vi "Check Finish Game.vi"(5 "Packed refs":T1, 7 "Game Result":refnum<vi>, 8 "error in (no error)":errorcluster, 11 "Board Game in":refnum<class "Board Game.lvclass">) -> (0 "error out":errorcluster, 1 "Finish Game?":bool, 3 "Board Game out":refnum<class "Board Game.lvclass">)   [LabVIEW 2021, in "Board Game.lvclass"]
uses:
  Board Game.lvclass
  Application/Packed Refs.ctl
  GameEl_class/private/Enum Direction.ctl
  Board Game.lvclass/Board Game.ctl
  Snake_class/Snake.lvclass/Snake.ctl
  GameEl_class/GameEl.lvclass/GameEl.ctl
  Imposible_Snake_v2/LVApp/Modules/Sound Manager/Typedefs/Sound Effects.ctl
  Game Result.ctl
  Snake_class/Read Bomb Crash.vi
  Snake_class/Read Star.vi
  GameEl_class/Read position.vi
  Snake_class/Read Snake Head.vi
  Snake_class/Snake.lvclass
  C:/Users/poche/Programs/LabVIEW/imposible snake/GameEl_class/GameEl.lvclass
  Imposible_Snake_v2/LVApp/Modules/Sound Manager/Sound Manager.lvlib
  GameEl_class/GameEl.lvclass
  Application/Game.lvclass
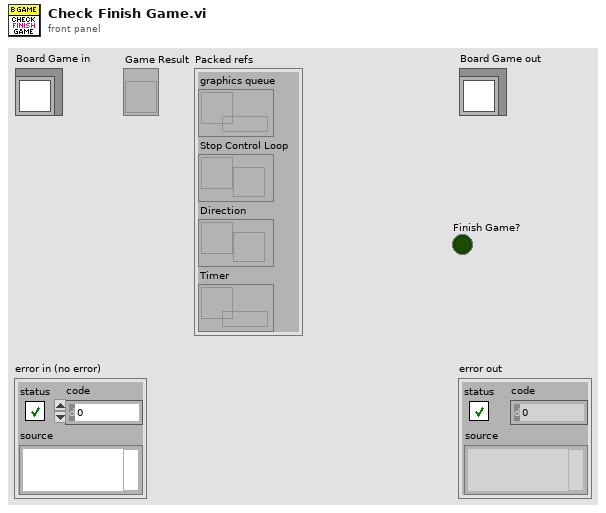
[diagram p1: front panel]
types:
  T1 = typedef "Game.lvclass/Packed Refs.ctl" = cluster{"graphics queue":refnum<queue>, "Stop Control Loop":refnum<user-event>, "Direction":refnum<notifier>, "Timer":refnum<data-value>}
  T2 = typedef "Sound Manager.lvlib/Sound Effects.ctl" = enum16{"Bomb In", "Bomb Out", "Bomb Touched", "Game Over", "Victory", "Eat", "10 Fruits", "Eat2", "Eat3", "Eat4", "MaxShield", "Shield", "10p", "Grape In", "Grape Out", "20p", "30p", "40p", "50p", "60p", "70p", "80p", "90p", "100p", "All shields cracked", "Mouse In", "Mouse Out", "Mouse Eaten", "Grape Eaten", "States Recover", "Broken Shield", "Bonus", "Happy Time", "explode", "Game over musica", "Back Music", "Shield Catch", "Evil lough", "Cricket In", "Cricket eaten", "Lets Go", "Jump1", "Jump2", "Jump3", "Unstoppable", "Troll Music", "winner", "menu"}
  T3 = typedef "Board Game.lvclass/Game Result.ctl" = enum16{"Game Over", "Game Finished", "Game Over - Bomb", "Game Over - Wall", "Game Over - Eat yourself"}
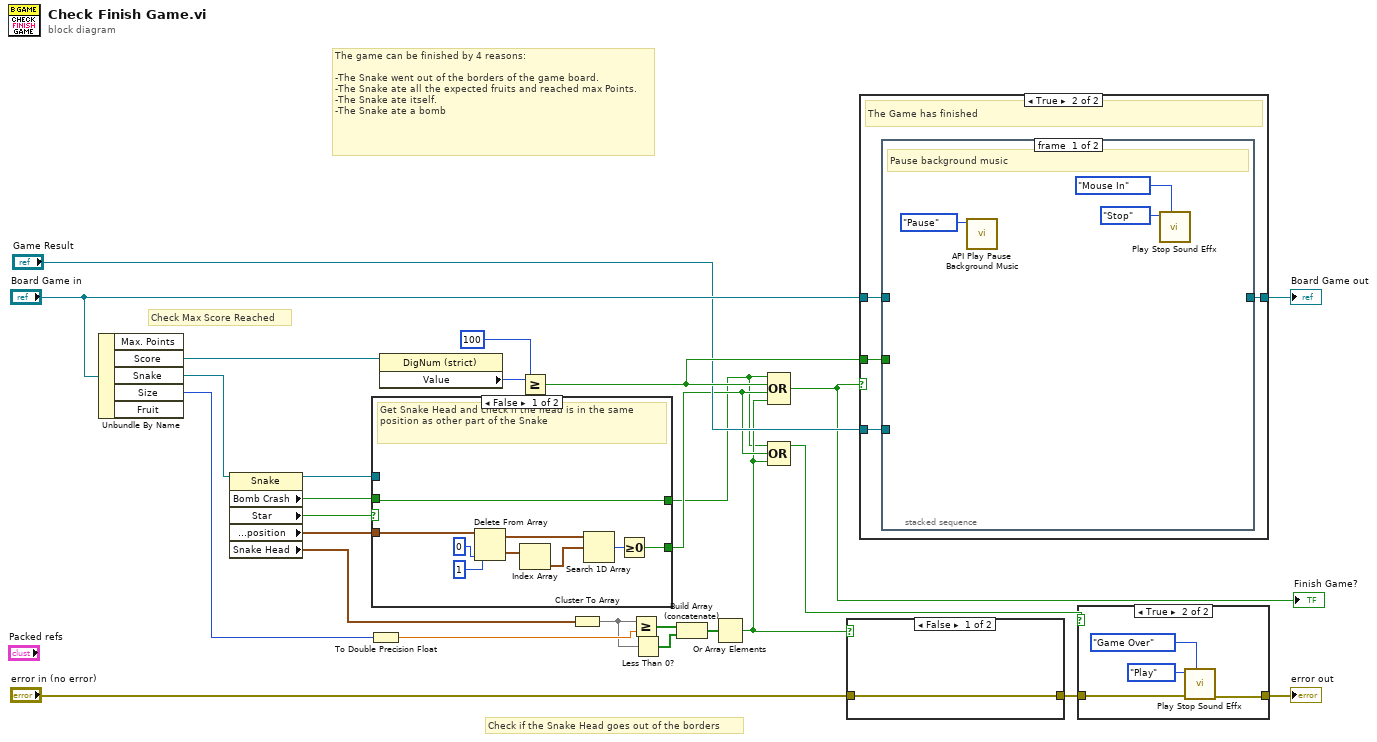
[diagram p0: block diagram]
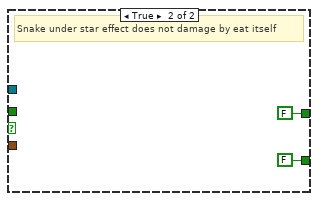
[diagram p2: hidden frame]
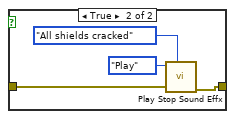
[diagram p3: hidden frame]
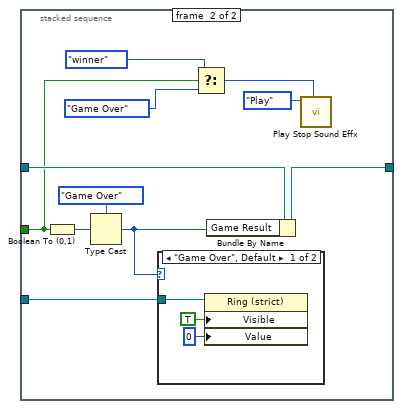
[diagram p6: hidden frame]
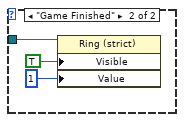
[diagram p7: hidden frame]
diagram:
  # "Check if the Snake Head goes out of the borders"
  # "Check Max Score Reached"
  # "The game can be finished by 4 reasons: \n\n-The Snake went out of the borders of the game board.\n-The Snake ate all the expected fruits and reached max Points.\n-The Snake ate itself. \n-The Snake ate a bomb"
  n1 = Unbundle By Name("Board Game in") -> ("Score"=w27:refnum<vi>, "Snake"=w25:refnum<class "Snake.lvclass">, "Size"=w24:u16)  [unwired: 2 out]
  n2 = property class="Snake"(reference=w25) -> (reference out=w7:refnum<class "Snake.lvclass">, "Bomb Crash"=w2:bool, "Star"=w6:bool, "SubVIs:DataAccess:position"=w5:cluster{"x":dbl, "y":dbl}[], "Snake Head"=w4:cluster{"x":dbl, "y":dbl})  [unwired: 1 in, 1 out]
  n3 = To Double Precision Float(number=w24) -> (double precision float=w23:dbl)
  n4 = case shown="False" w6 {
    tunnel: w7 -> [_ _]
    tunnel: [w30 FALSE] -> w12
    tunnel: w5 -> [w29 _]
    tunnel: w2 -> [w28 _]
    tunnel: [w28 FALSE] -> w1
    frame False {
      # "Get Snake Head and check if the head is in the same\nposition as other part of the Snake"
      n5 = Delete From Array(array=w29, length=1, index=0) -> (deleted portion=w34:cluster{"x":dbl, "y":dbl}[], array with subset deleted=w33:cluster{"x":dbl, "y":dbl}[])
      n6 = Index Array(array=w34) -> (element=w31:cluster{"x":dbl, "y":dbl})  [unwired: 1 in]
      n7 = Search 1D Array(1D array=w33, element=w31) -> (index of element=w32:i32)  [unwired: 1 in]
      n8 = Greater Or Equal To 0?(x=w32) -> (x >= 0?=w30:bool)
    }
    frame True {
      # "Snake under star effect does not damage by eat itself"
    }
  }
  n9 = property class="DigNum (strict)"(reference=w27) -> ("Value"=w26:u16)  [unwired: 1 in, 2 out]
  n10 = Greater Or Equal?(x=w26, y=u16 100) -> (x >= y?=w19:bool)
  n11 = Cluster To Array(cluster=w4) -> (array=w17:dbl[])
  n12 = Greater Or Equal?(x=w17, y=w23) -> (x >= y?=w22:bool[])
  n13 = Less Than 0?(x=w17) -> (x < 0?=w16:bool[])
  n14 = Build Array (concatenate)(w22, w16) -> (w18:bool[])
  n15 = Or Array Elements(Boolean array=w18) -> (logical OR=w8:bool)
  n16 = Compound Arithmetic op=OR(w1, w19, w12, w8) -> (w13:bool)
  "Finish Game?" <- w13
  n17 = Compound Arithmetic op=OR(w1, w12, w8) -> (w11:bool)
  n18 = case shown="False" w8 {
    tunnel: "error in (no error)" -> [w39 w41]
    tunnel: [w39 w40] -> w9
    frame False {
    }
    frame True {
      n19 = call "Play Stop Sound Effx.vi"("Sound Effect"=Sound_Effects."All shields cracked", "Error In"=w41, "Function"=enum16{"Play", "Stop"}."Play") -> ("error in (no error)"=w40:errorcluster)  [unwired: 8 in]
    }
  }
  n20 = case shown="True" w13 {
    tunnel: "Board Game in" -> [w44 w48]
    tunnel: [w44 w47] -> w20
    tunnel: w19 -> [_ w45]
    tunnel: "Game Result" -> [_ w46]
    frame False {
      # "The Game hasn't finished"
    }
    frame True {
      # "The Game has finished"
      n21 = stacked-sequence {
        tunnel: [_ w61] -> w47
        tunnel: w48 -> [_ w62]
        tunnel: w46 -> [_ w58]
        tunnel: w45 -> [_ w56]
        frame #0 {
          # "Pause background music"
          n22 = call "API Play Pause Background Music.vi"("Function"=enum16{"Pause", "Resume"}."Pause") -> ()  [unwired: 10 in, 1 out]
          n23 = call "Play Stop Sound Effx.vi"("Sound Effect"=Sound_Effects."Mouse In", "Function"=enum16{"Play", "Stop"}."Stop") -> ()  [unwired: 9 in, 1 out]
        }
        frame #1 {
          n24 = Boolean To (0,1)(Boolean=w56) -> (0, 1=w59:i16)
          n25 = Type Cast(type=Game_Result."Game Over" ("Game Result"), x=w59) -> (*(type *) &x=w57:T3)
          n26 = case shown="\"Game Over\", Default" w57 {
            tunnel: w58 -> [w64 w67]
            frame "Game Over", Default {
              n27 = property class="Ring (strict)"(reference=w64, "Visible"=TRUE, "Value"=u16 0) -> ()  [unwired: 1 in, 2 out]
            }
            frame "Game Finished" {
              n28 = property class="Ring (strict)"(reference=w67, "Visible"=TRUE, "Value"=u16 1) -> ()  [unwired: 1 in, 2 out]
            }
          }
          n29 = Select(t=Sound_Effects."winner" ("Sound Effect"), s=w56, f=Sound_Effects."Game Over") -> (s? t:f=w52:T2)
          n30 = Bundle By Name(cluster=w62, "Game Result"=w57) -> (w61:refnum<class "Board Game.lvclass">)
          n31 = call "Play Stop Sound Effx.vi"("Sound Effect"=w52, "Function"=enum16{"Play", "Stop"}."Play") -> ()  [unwired: 9 in, 1 out]
        }
      }
    }
  }
  "Board Game out" <- w20
  n32 = case shown="True" w11 {
    tunnel: w9 -> [w69 w71]
    tunnel: [w69 w70] -> w14
    frame False {
    }
    frame True {
      n33 = call "Play Stop Sound Effx.vi"("Sound Effect"=Sound_Effects."Game Over", "Error In"=w71, "Function"=enum16{"Play", "Stop"}."Play") -> ("error in (no error)"=w70:errorcluster)  [unwired: 8 in]
    }
  }
  "error out" <- w14
